vi "ICNC MB Control.vi"(8 "error in (no error)":errorcluster caption="entrée d'erreur (pas d'erreur)", 10 "ptBuffer":string, 11 "SubCommandID":i32) -> (0 "error out":errorcluster caption="sortie d'erreur", 2 "ptBuffer out":string, 3 "function return":u32)   [LabVIEW 2012, in "ICNC2.lvlib"]
doc: "DWORD ICNC_MBControl ( int SubCommandID,\n unsigned char *ptBuffer);"
uses:
  <userlib>/ICNC/ICNC2.lvlib
  <userlib>/ICNC/ICNC2.dll
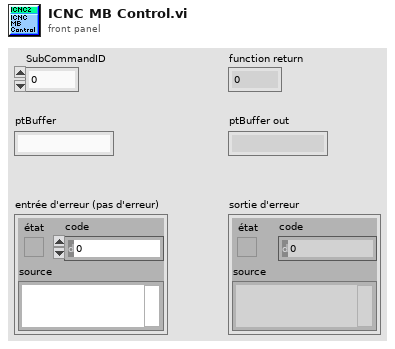
[diagram p1: front panel]
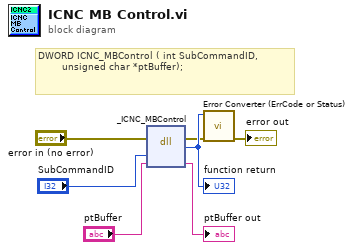
[diagram p0: block diagram]
diagram:
  # "DWORD ICNC_MBControl ( int SubCommandID,\n\t\t\t\t\t   unsigned char *ptBuffer);"
  n1 = dll-call lib="C:/Program Files (x86)/National Instruments/LabVIEW 2012/user.lib/ICNC/ICNC2.*" fn="_ICNC_MBControl"(error in="error in (no error)", "SubCommandID"="SubCommandID", "ptBuffer"="ptBuffer") -> (error out=w2:errorcluster, w7:u32, "ptBuffer"=→"ptBuffer out":string)  [unwired: 3 in, 1 out]
  "function return" <- w7
  n2 = call <userlib>:"Error Converter (ErrCode or Status).vi"("error in (no error)"=w2, "error code"=w7) -> ("error out"=→"error out":errorcluster)  [unwired: 9 in]
